vi "WFGDynamicConfigCh.vi"(0 "object in":refnum<class "AD2_WFG_SDK.lvclass">, 5 "error in (no error)":errorcluster) -> (14 "object out":refnum<class "AD2_WFG_SDK.lvclass">, 19 "error out":errorcluster)   [LabVIEW 2019, in "AD2_WFG_SDK.lvclass"]
uses:
  AD2_WFG_SDK.lvclass
  AD2_WFG_SDK.lvclass/AD2_WFG_SDK.ctl
  Olasdwf/Olasdwf.lvlib
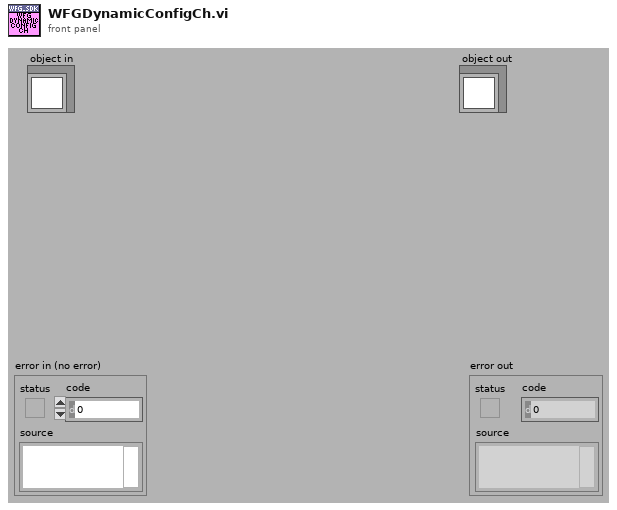
[diagram p1: front panel]
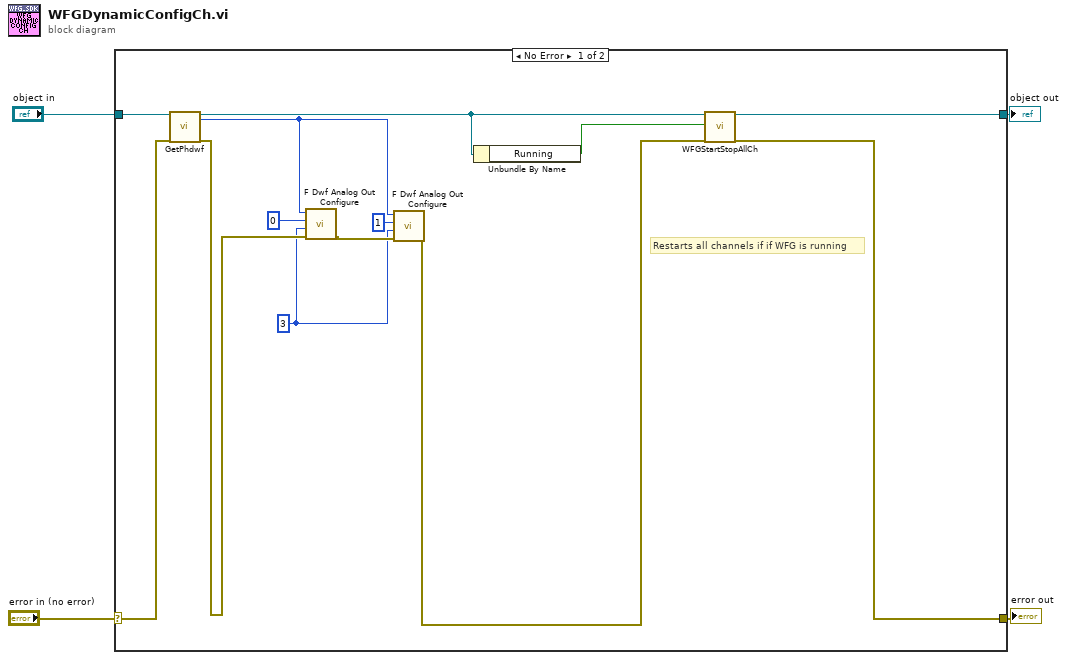
[diagram p0: block diagram]
diagram:
  n1 = case shown="No Error" "error in (no error)" {
    selector: "error in (no error)" -> [w17 w19]
    tunnel: [w7 w19] -> w3
    tunnel: [w9 w18] -> w1
    tunnel: "object in" -> [w16 w18]
    frame No Error {
      w12 = 3 ("fStart")
      # "Restarts all channels if if WFG is running"
      n2 = call-dynamic "GetPhdwf.vi"("object in"=w16, "error in (no error)"=w17) -> ("object out"=w6:refnum<class "AD2_WFG_SDK.lvclass">, "phdwf"=w13:i32, "error out"=w15:errorcluster)  [unwired: 15 in]
      n3 = call "F Dwf Analog Out Configure.vi"("error in (no error)"=w15, "fStart"=w12, "idxChannel"=0, "hdwf"=w13) -> ("error out"=w14:errorcluster)  [unwired: 6 in, 1 out]
      n4 = call "F Dwf Analog Out Configure.vi"("error in (no error)"=w14, "fStart"=w12, "idxChannel"=1, "hdwf"=w13) -> ("error out"=w8:errorcluster)  [unwired: 6 in, 1 out]
      n5 = Unbundle By Name(w6) -> ("Running"=w5:bool)
      n6 = call-dynamic "WFGStartStopAllCh.vi"("object in"=w6, "Start"=w5, "error in (no error)"=w8) -> ("object out"=w9:refnum<class "AD2_WFG_SDK.lvclass">, "error out"=w7:errorcluster)  [unwired: 15 in]
    }
    frame Error {
    }
  }
  "error out" <- w3
  "object out" <- w1
